vi "single channel close_open.vi"(2 "error in":T1, 3 "channel":i16=1, 4 "open all 0 / close 2":i16, 5 "VISA resource name":refnum<visa-resource-name>="GPIB0::10::INSTR") -> (0 "error out":T1)   [LabVIEW 2019]
uses:
  <instrlib>/ke7001/KE7001.LLB/Keith 7001 Open/Close Chan.vi
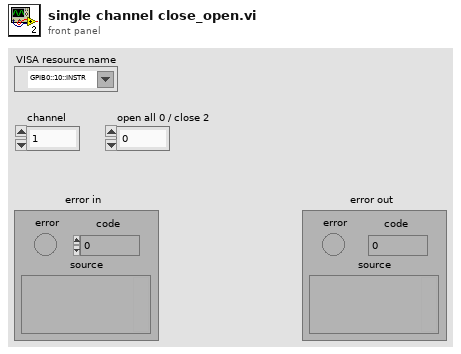
[diagram p1: front panel]
types:
  T1 = cluster{"error":bool, "code":i32, "source":string}
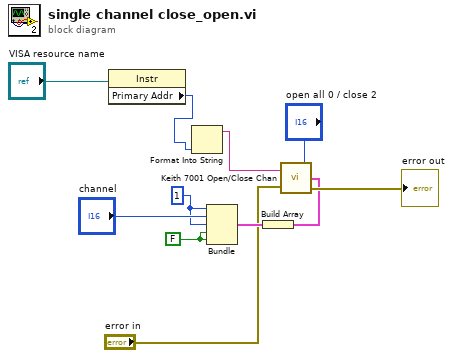
[diagram p0: block diagram]
diagram:
  w7 = 1
  w9 = FALSE
  n1 = property class="Instr"(reference="VISA resource name") -> ("Primary Addr"=w2:u16)  [unwired: 1 in, 2 out]
  n2 = Format Into String(w2) -> (resulting string=w4:string)  [unwired: 3 in, 1 out]
  n3 = Bundle(w7, "channel"="channel", w7, w9, w9) -> (w6:cluster{i32, "channel":i16, i32, bool, bool})  [unwired: 1 in]
  n4 = Build Array(w6) -> (w5:cluster{i32, "channel":i16, i32, bool, bool}[])
  n5 = call "Keith 7001 Open/Close Chan.vi"("GPIB address"=w4, "error in"="error in", "open/close (open all:0)"="open all 0 / close 2", "channel list"=w5) -> ("error out"=→"error out":T1)
